vi "ROI entry-Get last event.vi"(8 "error in (no error)":errorcluster) -> (0 "error out":errorcluster, 2 "Type":i32(ring) items=["No Event"=0, "Click Event"=1, "Draw Event"=2, "Size Event"=4, "Scroll Event"=5, "Double Click Event"=8], 3 "Last Image Display Event info":T1 {"Tool" items=["None", "Selection Tool", "Point Tool", "Line Tool", "Rectangle Tool", "Oval Tool", "Polygon Tool", "ClosedFreehandTool", "Annulus Tool", "Rotated Rectangle Tool", "Zoom Tool", "Pan Tool", "Polyline Tool", "Freehand Tool"]; "Type" items=["No Event"=0, "Click Event"=1, "Draw Event"=2, "Size Event"=4, "Scroll Event"=5, "Double Click Event"=8]})   [LabVIEW 2017]
uses:
  Typedefs/Last Image Display Event info.ctl
  ROI Entry screen/Globals/gl_ROI Entry UI globals.vi
panel:
  out "Tool":i32(ring) items=["None", "Selection Tool", "Point Tool", "Line Tool", "Rectangle Tool", "Oval Tool", "Polygon Tool", "ClosedFreehandTool", "Annulus Tool", "Rotated Rectangle Tool", "Zoom Tool", "Pan Tool", "Polyline Tool", "Freehand Tool"]
  out "Coordinates":i32[](array[numeric])
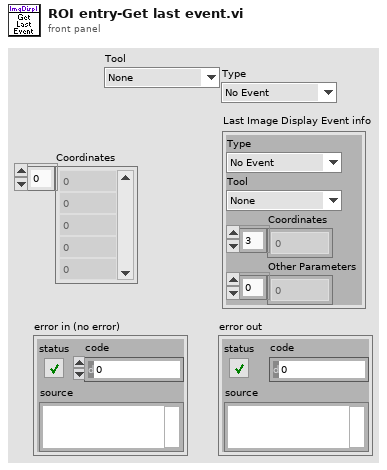
[diagram p1: front panel]
types:
  T1 = typedef "Last Image Display Event info.ctl" = cluster{"Type":i32, "Tool":i32, "Coordinates":i32[], "Other Parameters":sgl[]}
  T2 = cluster{"Type":i32, "Tool":i32, "Coordinates":i32[], "Other Parameters":sgl[]}
  T3 = typedef "ROI entry screen ctrl refs cluster.ctl" = cluster{"Done button":refnum<vi>, "Imaging button":refnum<vi>, "Acquisition button":refnum<vi>, "POI dwell time (us)":refnum<vi>, "Scan dwell time per pixel (us)":refnum<vi>, "# of planes":refnum<vi>, "Zoom Ctrl":refnum<vi>, "Equal size":refnum<vi>, "Channel":refnum<vi>, "Image Display":refnum<vi>, "Z-Plane Selector":refnum<vi>, "Number of lines left":refnum<vi>, "Z-stack folder path":refnum<vi>, "POI Density":refnum<vi>, "Arb Plane Entry":refnum<vi>, "Whole plane":refnum<vi>, "Clear Last":refnum<vi>, "Clear All":refnum<vi>, "Trial Length (sec)":refnum<vi>, "Palette Type":refnum<vi>, "Intensity slider":refnum<vi>, "# POI":refnum<vi>, "Max Z Proj":refnum<vi>, "Zplane ind":refnum<vi>, "Wavelength (nm)":refnum<vi>, "Number of Trials":refnum<vi>, "Funct stim.trig.enable":refnum<vi>, "Funct stim.trig.delay (s)":refnum<vi>, "Line Mode":refnum<vi>, "Step size (µm)":refnum<vi>, "ROI move mode":refnum<vi>, "Cool-down time (s)":refnum<vi>, "Enable cool-down time":refnum<vi>, "Motor Z ind. (um)":refnum<vi>, "AOL Z ind. (um)":refnum<vi>, "Load Reference Image":refnum<vi>}
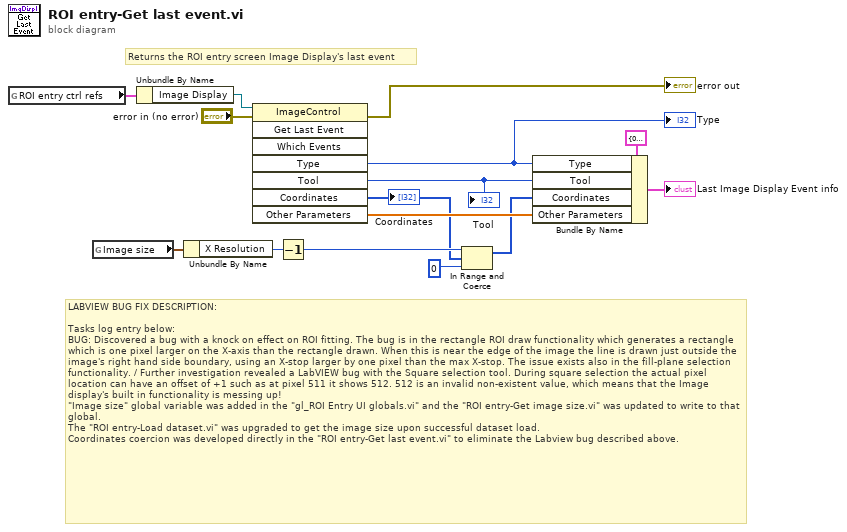
[diagram p0: block diagram]
diagram:
  # "LABVIEW BUG FIX DESCRIPTION:\n\nTasks log entry below:\nBUG: Discovered a bug with a knock on effect on ROI fitting. The bug is in the rectangle ROI draw functionality which generates a rectangle which is one pixel larger on the X-axis than the rectangle drawn. When this is near the edge of the image the line is drawn just outside the image's right hand side boundary, using an X-stop larger by one pixel than the max X-stop. The issue exists also in the fill-plane selection functionality. / Further investigation revealed a LabVIEW bug with the Square selection tool. During square selection the actual pixel location can have an offset of +1 such as at pixel 511 it shows 512. 512 is an invalid non-existent value, which means that the Image display's built in functionality is messing up!\n\"Image size\" global variable was added in the \"gl_ROI Entry UI globals.vi\" and the \"ROI entry-Get image size.vi\" was updated to write to that global.\nThe \"ROI entry-Load dataset.vi\" was upgraded to get the image size upon successful dataset load.\nCoordinates coercion was developed directly in the \"ROI entry-Get last event.vi\" to eliminate the Labview bug described above."
  # "Returns the ROI entry screen Image Display's last event"
  n1 = global read "gl_ROI Entry UI globals.vi" "ROI entry ctrl refs"() -> (w15:T3)
  n2 = global read "gl_ROI Entry UI globals.vi" "Image size"() -> (w6:cluster{"X Resolution":i32, "Y Resolution":i32})
  n3 = Unbundle By Name(w15) -> ("Image Display"=w14:refnum<vi>)
  n4 = Unbundle By Name(w6) -> ("X Resolution"=w5:i32)
  n5 = invoke on="Invoke Node" class="ImageControl" method="Get Last Event"(reference=w14, error in="error in (no error)") -> (error out=→"error out":errorcluster, "Type"=w7:i32, "Tool"=w10:i32, "Coordinates"=w1:i32[], "Other Parameters"=w9:sgl[])  [unwired: 6 in, 3 out]
  "Type" <- w7
  "Coordinates" <- w1
  "Tool" <- w10
  n6 = Decrement(x=w5) -> (x-1=w4:i32)
  n7 = In Range and Coerce(upper limit=w4, x=w1, lower limit=0 ("x-1")) -> (coerced(x)=w2:i32[])  [unwired: 1 out]
  n8 = Bundle By Name(cluster=T2 {"Type"=0, "Tool"=0, "Coordinates"=[], "Other Parameters"=[]} ("Cluster"), "Type"=w7, "Tool"=w10, "Coordinates"=w2, "Other Parameters"=w9) -> (→"Last Image Display Event info":T2)
